vi "AR Drone - Gamepad NavData Video.vi"() -> ()   [LabVIEW 2014]
doc: "Example demonstrating how to control the AR Drone with a joystick or gamepad and simultaneously receive navigation and video data."
uses:
  <vilib>/LVH/AR Drone Toolkit/Decode NavData/Typedefs/NavData Demo.ctl
  <vilib>/LVH/AR Drone Toolkit/Type Defs/Flight Animations.ctl
  <vilib>/Utility/inputDevices.llb/closeJoystick.vi
  <vilib>/LVH/AR Drone Toolkit/AR Drone.lvlib
panel:
  out "Gamepad Output":T1
  in  "Flight Animations":T2 items=["PHI_M30_DEG", "PHI_30_DEG", "THETA_M30_DEG", "THETA_30_DEG", "THETA_20DEG_YAW_200DEG", "THETA_20DEG_YAW_M2000DEG", "TURNAROUND", "TURNAROUND_GODOWN", "YAW_SHAKE", "YAW_DANCE", "PHI_DANCE", "THETA_DANCE", "VZ_DANCE", "WAVE", "PHI_THETA_MIXED", "DOUBLE_PHI_THETA_MIXED", "FLIP_AHEAD", "FLIP_BEHIND", "FLIP_LEFT", "FLIP_RIGHT", "NB_ANIM_MAYDAY"]
  out "Video Stream":picture
  out "NavData Out":T3
  out "Battery Remaining":dbl(slide) scale=0.0..100.0
  out "Axes Output":T4 {"Vertical Speed" scale=-1.0..1.0; "Yaw Speed" scale=-1.0..1.0; "Pitch" scale=-1.0..1.0; "Roll" scale=-1.0..1.0}
  in  "stop":bool
  # "Xbox Controller:\nLeft stick L/R - Roll\nLeft stick D/U - Pitch\nL/R Triggers - Vertical Speed\nRight stick L/R - Yaw Speed"
  # "Xbox Controller:\nA - take off\nB - emergency\nX - hover\nStart - Stop"
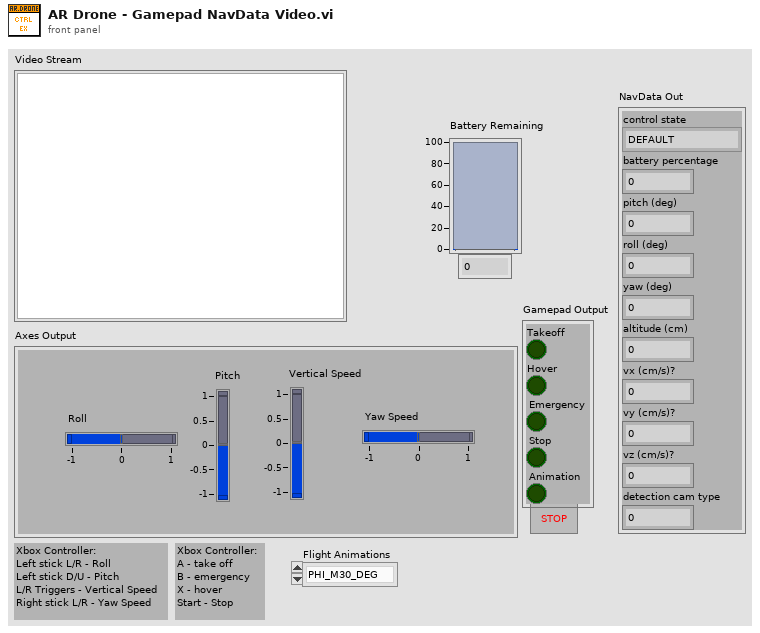
[diagram p1: front panel]
types:
  T1 = cluster{"Takeoff":bool, "Hover":bool, "Emergency":bool, "Stop":bool, "Animation":bool}
  T2 = typedef "AR Drone.lvlib/Flight Animations.ctl" = u16
  T3 = typedef "AR Drone.lvlib/NavData Demo.ctl" = cluster{"control state":enum32{"DEFAULT", "INIT", "LANDING", "FLYING", "HOVERING", "TEST", "TRANS_TAKEOFF", "TRANS_GOTOFIX", "TRANS_LANDING"}, "battery percentage":u32, "pitch (deg)":sgl, "roll (deg)":sgl, "yaw (deg)":sgl, "altitude (cm)":u32, "vx (cm/s)?":sgl, "vy (cm/s)?":sgl, "vz (cm/s)?":sgl, "detection cam type":u32}
  T4 = cluster{"Roll":dbl, "Pitch":dbl, "Vertical Speed":dbl, "Yaw Speed":dbl}
  T5 = typedef "AR Drone.lvlib/AR Drone Resource.ctl" = cluster{"UDP Control Connection":refnum<k16>, "UDP NavData Connection":refnum<k16>, "UDP Video Connection (Drone 1.0)":refnum<k16>, "TCP Video Connection (Drone 2.0)":refnum<k5>, "TCP Control Port Connection":refnum<k5>, "Drone IP address":string, "Drone Command Port":u16, "Drone NavData Port":u16, "Drone Vid Stream Port":u16, "Drone TCP Control Port":u16, "Home IP address":string, "Home Command Port":u16, "Home NavData Port":u16, "Home Vid Stream Port":u16, "Drone Version":i32}
  T6 = cluster{"Roll":sgl, "Pitch":sgl, "Vertical Speed":sgl, "Yaw Speed":sgl}
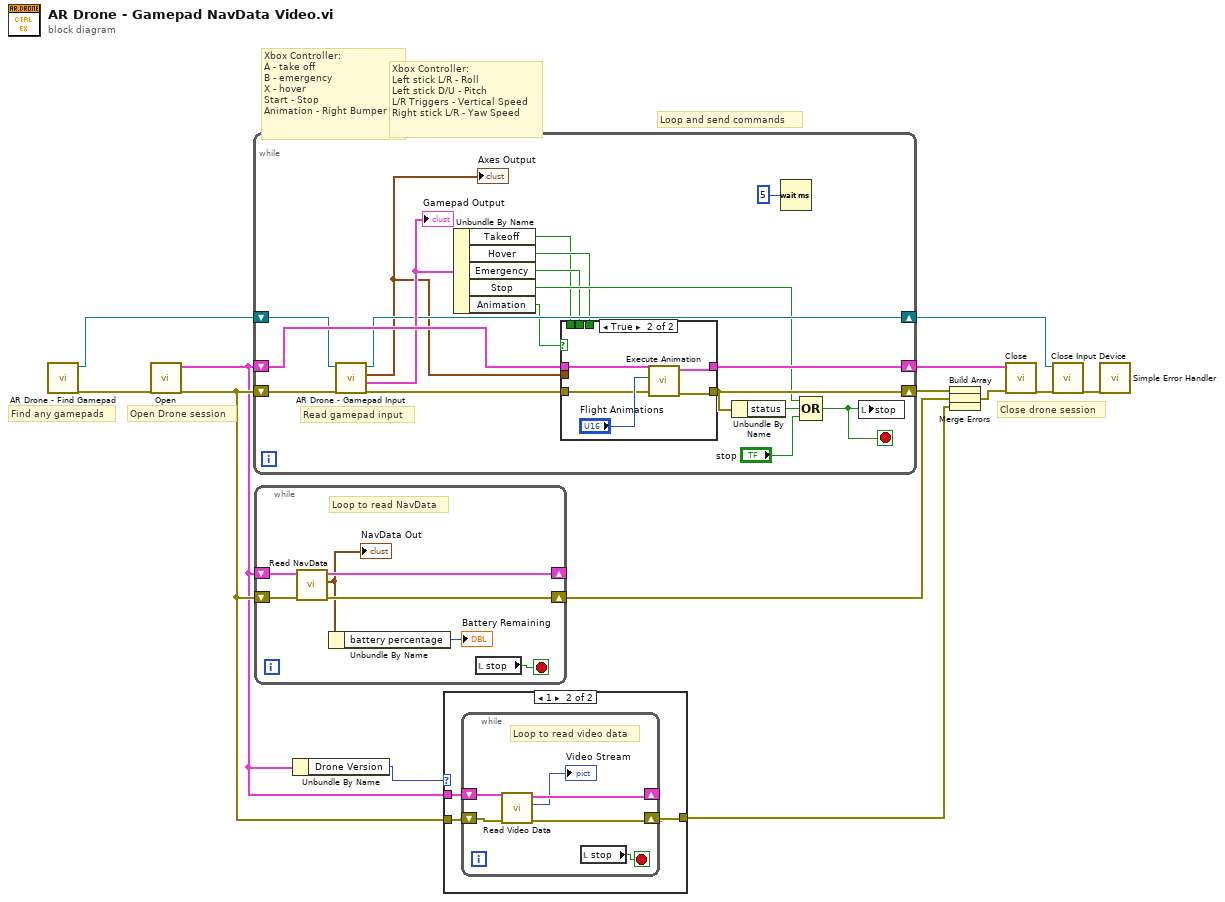
[diagram p0: block diagram]
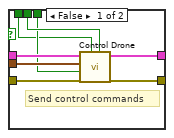
[diagram p3: hidden frame]
diagram:
  # "Loop and send commands"
  # "Close drone session"
  # "Open Drone session"
  # "Find any gamepads"
  # "Xbox Controller:\nLeft stick L/R - Roll\nLeft stick D/U - Pitch\nL/R Triggers - Vertical Speed\nRight stick L/R - Yaw Speed"
  # "Xbox Controller:\nA - take off\nB - emergency\nX - hover\nStart - Stop\nAnimation - Right Bumper"
  n1 = call "AR Drone - Find Gamepad.vi"() -> ("error out"=w9:errorcluster, "Refnum out"=w10:refnum<k1>)  [unwired: 10 in]
  n2 = call <vilib>:"Open.vi"("error in (no error)"=w9) -> ("error out"=w4:errorcluster, "AR Drone Resource"=w2:T5)  [unwired: 9 in]
  n3 = while {
    shift-right: [w31] -> w14
    shift-left: w2 -> [w32]
    shift-right: [w30] -> w7
    shift-left: w4 -> [w25]
    shift-right: [w22] -> w13
    shift-left: w10 -> [w26]
    stop <- w16 stop-if-true
    # "Read gamepad input"
    n4 = call "AR Drone - Gamepad Input.vi"("error in (no error)"=w25, "Refnum in"=w26) -> ("error out"=w24:errorcluster, "Gamepad Output"=w23:T1, "Control Cluster"=w21:T6, "Refnum out"=w22:refnum<k1>)  [unwired: 6 in]
    "Axes Output" <- w21
    "Gamepad Output" <- w23
    n5 = Unbundle By Name(w23) -> ("Takeoff"=w17:bool, "Hover"=w18:bool, "Emergency"=w19:bool, "Stop"=w20:bool, "Animation"=w15:bool)
    n6 = case shown="True" w15 {
      tunnel: w32 -> [w40 w43]
      tunnel: [w39 w41] -> w31
      tunnel: [w38 w42] -> w30
      tunnel: w24 -> [w37 w44]
      tunnel: w21 -> [w36 _]
      tunnel: w19 -> [w35 _]
      tunnel: w18 -> [w34 _]
      tunnel: w17 -> [w33 _]
      frame False {
        # "Send control commands"
        n7 = call <vilib>:"Control Drone.vi"("Emergency Landing"=w35, "Takeoff/Land"=w33, "error in (no error)"=w37, "Hover"=w34, "Control Cluster"=w36, "AR Drone Resource"=w40) -> ("error out"=w38:errorcluster, "AR Drone Resource Out"=w39:T5)  [unwired: 4 in]
      }
      frame True {
        n8 = call <vilib>:"Execute Animation.vi"("error in (no error)"=w44, "Flight Animation"="Flight Animations", "AR Drone Resource"=w43) -> ("error out"=w42:errorcluster, "AR Drone Resource Out"=w41:T5)  [unwired: 7 in]
      }
    }
    n9 = Unbundle By Name(w30) -> ("status"=w28:bool)
    n10 = Wait (ms)(milliseconds to wait=u32 5) -> ()  [unwired: 1 out]
    n11 = Compound Arithmetic op=OR(w20, w28, "stop") -> (w16:bool)
    n12 = local write "stop"(w16) -> ()
  }
  n13 = while {
    shift-right: [w51] -> _
    shift-left: w2 -> [w52]
    shift-right: [w49] -> w6
    shift-left: w4 -> [w50]
    stop <- w46 stop-if-true
    # "Loop to read NavData"
    n14 = call <vilib>:"Read NavData.vi"("error in (no error)"=w50, "AR Drone Resource"=w52) -> ("error out"=w49:errorcluster, "NavData Out"=w48:T3, "AR Drone Resource Out"=w51:T5)  [unwired: 7 in]
    "NavData Out" <- w48
    n15 = Unbundle By Name(w48) -> ("battery percentage"=→"Battery Remaining":u32)
    n16 = local read "stop"() -> (w46:bool)
  }
  n17 = Unbundle By Name(w2) -> ("Drone Version"=w1:i32)
  n18 = case shown="1" w1 {
    tunnel: w2 -> [_ w56]
    tunnel: [w53 w55] -> w5
    tunnel: w4 -> [w53 w54]
    frame 2, Default {
      # "If Drone 2.0, no streaming in line"
    }
    frame 1 {
      n19 = while {
        shift-right: [w60] -> _
        shift-left: w56 -> [w62]
        shift-right: [w59] -> w55
        shift-left: w54 -> [w61]
        stop <- w57 stop-if-true
        # "Loop to read video data"
        n20 = call <vilib>:"Read Video Data.vi"("error in (no error)"=w61, "AR Drone Resource"=w62) -> ("error out"=w59:errorcluster, "Video Stream"=→"Video Stream":picture, "AR Drone Resource Out"=w60:T5)  [unwired: 7 in]
        n21 = local read "stop"() -> (w57:bool)
      }
    }
  }
  n22 = Build Array(w7, w6, w5) -> (w3:errorcluster[])
  n23 = Merge Errors(w3) -> (w8:errorcluster)
  n24 = call <vilib>:"Close.vi"("error in (no error)"=w8, "AR Drone Resource"=w14) -> ("error out"=w12:errorcluster)  [unwired: 9 in]
  n25 = call-poly <vilib>:"Close Input Device.vi"("error in (no error)"=w12, "device ID"=w13) -> ("error out"=w11:errorcluster)  [unwired: 8 in]
  n26 = call <vilib>:"Simple Error Handler.vi"("error in (no error)"=w11) -> ()  [unwired: 4 in, 5 out]
